vi "TWM Wait for Measure End.vi"(0 "handle":i32, 1 "end of packet key":string="TWM:command:EndOfPacket", 2 "Obtain results? (False)":bool, 3 "timeout [s] (10s)":dbl=30.0, 5 "meas root path (last)":path, 7 "quantity names (all)":string[](array[string]), 9 "stop ref (none)":refnum<vi>, 11 "error in":errorcluster, 12 "qwtb maxdim (scalar)":T3 caption="Max. shown dimension (scalar)", 13 "status ref (none)":refnum<vi>, 14 "phase ref channel tag (none)":string) -> (4 "handle out":i32, 6 "data":T2[][](array[typedef]), 8 "stoped?":bool, 10 "quantities":T1, 15 "error out":errorcluster)   [LabVIEW 2020]
doc: "TWM client top level function: Start measurement, wait for completion, Get result.\n\nSet reasonable timeout for the TWM sampling and processing. Wire in the the 'stop' reference to allow termination of the TWM task."
uses:
  external libraries/TWM client/TWM Client Result Max Dim.ctl
  external libraries/TWM client/TWM Client Quantity Record.ctl
  external libraries/TWM client/TWM Client Result Info.ctl
  <vilib>/Utility/error.llb/Error Cluster From Error Code.vi
  <vilib>/ErrorRing/Error Ring.xnode
  external libraries/TWM client/TWM Client.lvlib
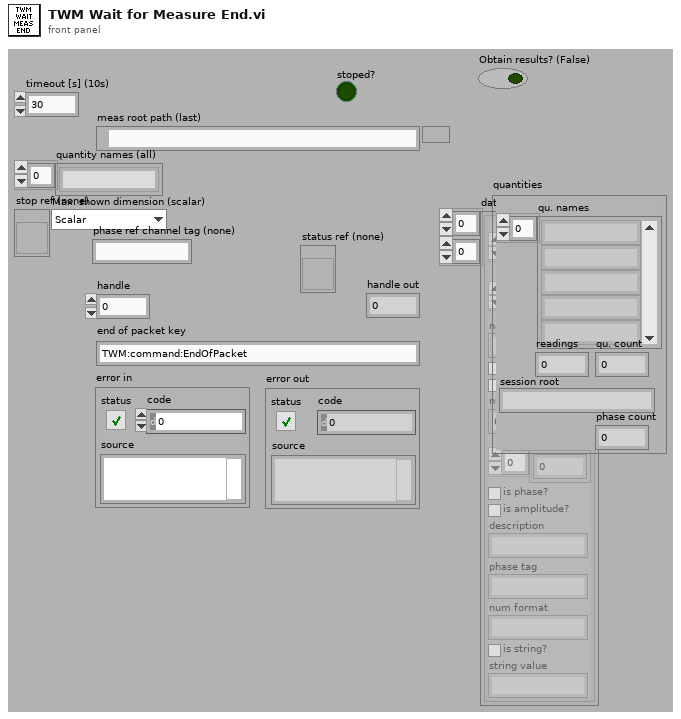
[diagram p1: front panel]
types:
  T1 = typedef "TWM Client.lvlib/TWM Client Result Info.ctl" = cluster{"qu. names":string[], "readings":i32, "qu. count":i32, "session root":string, "phase count":i32}
  T2 = typedef "TWM Client.lvlib/TWM Client Quantity Record.ctl" = cluster{"val":dbl[], "unc":dbl[], "name":string, "is valid?":bool, "has unc?":bool, "numel":i32, "ua":dbl[], "is phase?":bool, "is amplitude?":bool, "description":string, "phase tag":string, "num format":string, "is string?":bool, "string value":string}
  T3 = typedef "TWM Client.lvlib/TWM Client Result Max Dim.ctl" = enum16{"Scalar", "Vector", "Matrix"}
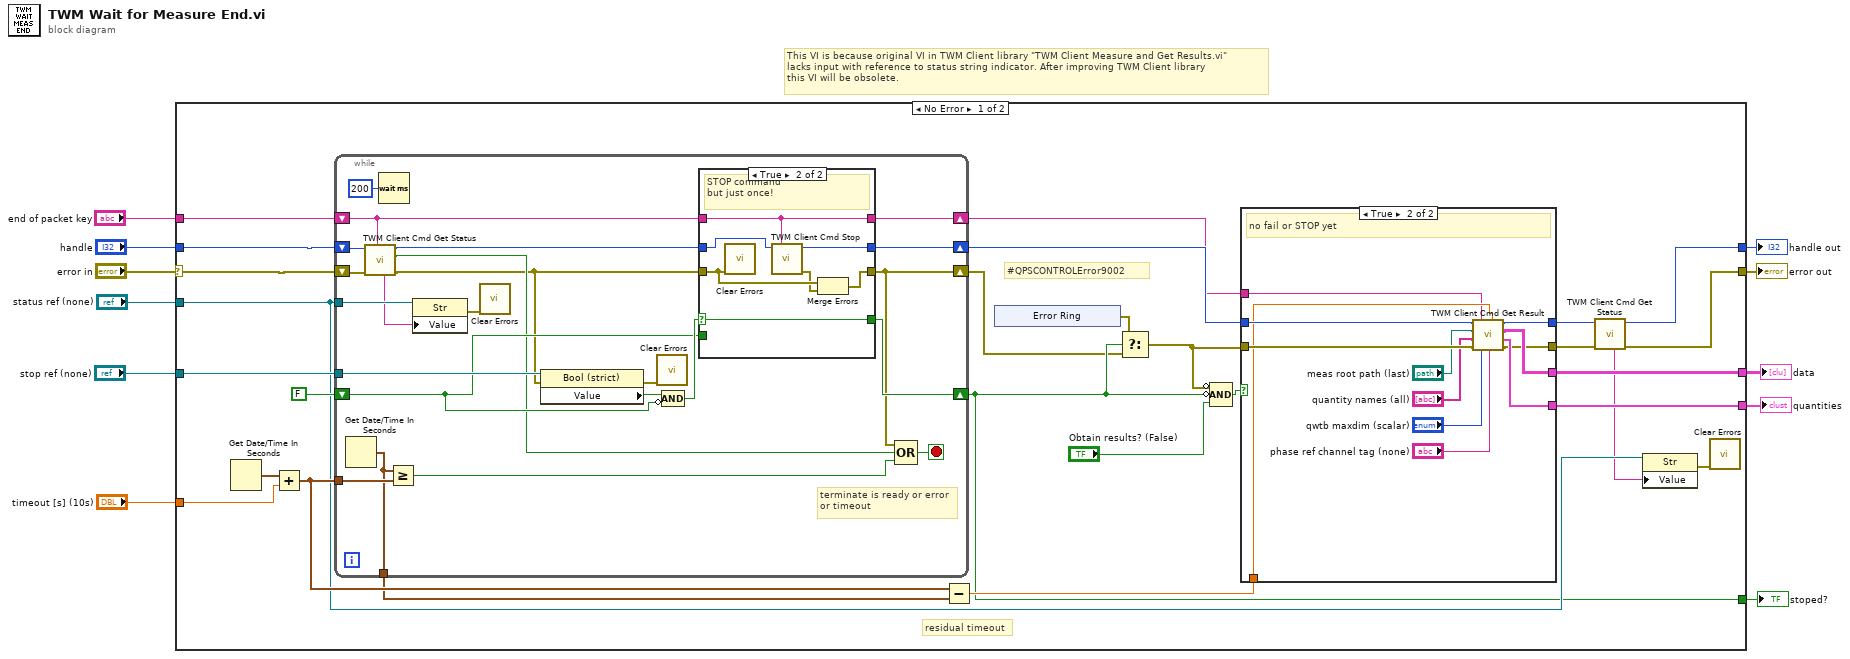
[diagram p0: block diagram]
diagram:
  # "This VI is because original VI in TWM Client library \"TWM Client Measure and Get Results.vi\"\nlacks input with reference to status string indicator. After improving TWM Client library \nthis VI will be obsolete."
  n1 = case shown="No Error" "error in" {
    selector: "error in" -> [w14 w93]
    tunnel: "handle" -> [w13 w92]
    tunnel: "stop ref (none)" -> [w38 _]
    tunnel: "timeout [s] (10s)" -> [w36 _]
    tunnel: "end of packet key" -> [w26 _]
    tunnel: [w24 w92] -> w7
    tunnel: [w22 w93] -> w6
    tunnel: [w28 _] -> w5
    tunnel: [w27 _] -> w4
    tunnel: [w18 _] -> w2
    tunnel: "status ref (none)" -> [w20 _]
    frame No Error {
      # "#QPSCONTROLError9002"
      # "residual timeout"
      n2 = Get Date/Time In Seconds() -> (seconds since 1Jan1904=w35:timestamp)
      n3 = Add(x=w35, y=w36) -> (x+y=w34:timestamp)
      n4 = while {
        shift-right: [w78] -> w31
        shift-left: w13 -> [w62]
        shift-right: [w72] -> w16
        shift-left: w14 -> [w63]
        tunnel: w38 -> [w79]
        shift-right: [w77] -> w18
        shift-left: FALSE -> [w74]
        tunnel: w34 -> [w73]
        tunnel: [w68] -> w33
        shift-right: [w67] -> w29
        shift-left: w26 -> [w61]
        tunnel: w20 -> [w60]
        stop <- w70 stop-if-true
        # "terminate is ready or error\nor timeout"
        n5 = Get Date/Time In Seconds() -> (seconds since 1Jan1904=w68:timestamp)
        n6 = call "TWM Client Cmd Get Status.vi"("end of packet key"=w61, "error in"=w63, "handle"=w62) -> ("error out"=w64:errorcluster, "ready?"=w65:bool, "handle out"=w66:i32, "status string"=w59:string)  [unwired: 4 in, 1 out]
        n7 = Wait (ms)(milliseconds to wait=u32 200) -> ()  [unwired: 1 out]
        n8 = Greater Or Equal?(x=w68, y=w73) -> (x >= y?=w71:bool)
        n9 = property class="Str"(reference=w60, "Value"=w59) -> (error out=w58:errorcluster)  [unwired: 1 in, 1 out]
        n10 = call <vilib>:"Clear Errors.vi"("error in (no error)"=w58) -> ()  [unwired: 5 in, 2 out]
        n11 = property class="Bool (strict)"(reference=w79, error in=w64) -> (error out=w80:errorcluster, "Value"=w76:bool)  [unwired: 1 out]
        n12 = call <vilib>:"Clear Errors.vi"("error in (no error)"=w80) -> ()  [unwired: 5 in, 2 out]
        n13 = Compound Arithmetic op=AND(w76, invert w74) -> (w75:bool)
        n14 = case shown="True" w75 {
          selector: w75 -> [_ w89]
          tunnel: w64 -> [w84 w91]
          tunnel: w66 -> [w83 w86]
          tunnel: [w83 w88] -> w78
          tunnel: [w84 w90] -> w72
          tunnel: [w82 w89] -> w77
          tunnel: w74 -> [w82 _]
          tunnel: w61 -> [w81 w87]
          tunnel: [w81 w87] -> w67
          frame False {
          }
          frame True {
            # "STOP command\nbut just once!"
            n15 = call <vilib>:"Clear Errors.vi"("error in (no error)"=w91) -> ()  [unwired: 5 in, 2 out]
            n16 = call "TWM Client Cmd Stop.vi"("end of packet key"=w87, "handle"=w86) -> ("error out"=w85:errorcluster, "handle out"=w88:i32)  [unwired: 8 in]
            n17 = Merge Errors(w91, w85) -> (w90:errorcluster)
          }
        }
        n18 = Compound Arithmetic op=OR(w72, w65, w71) -> (w70:bool)
      }
      n19 = Subtract(x=w34, y=w33) -> (x-y=w30:dbl)
      n20 = xnode "Error Ring"() -> ("error out"=w15:errorcluster)
      n21 = Select(t=w15, s=w18, f=w16) -> (s? t:f=w17:errorcluster)
      n22 = Compound Arithmetic op=AND(invert w17, invert w18, "Obtain results? (False)") -> (w32:bool)
      n23 = case shown="True" w32 {
        tunnel: w17 -> [w45 w52]
        tunnel: w31 -> [w44 w57]
        tunnel: [w45 w53] -> w23
        tunnel: [w44 w56] -> w25
        tunnel: w30 -> [_ w51]
        tunnel: w29 -> [_ w50]
        tunnel: [_ w55] -> w28
        tunnel: [_ w54] -> w27
        frame False {
          # "STOP or error"
        }
        frame True {
          # "no fail or STOP yet"
          n24 = call "TWM Client Cmd Get Result.vi"("phase ref channel tag (none)"="phase ref channel tag (none)", "timeout [s] (10s)"=w51, "qwtb maxdim (scalar)"="qwtb maxdim (scalar)", "end of packet key"=w50, "error in"=w52, "quantity names (all)"="quantity names (all)", "meas root path (last)"="meas root path (last)", "handle"=w57) -> ("error out"=w53:errorcluster, "result info"=w54:T1, "result data"=w55:T2[][], "handle out"=w56:i32)
        }
      }
      n25 = call "TWM Client Cmd Get Status.vi"("error in"=w23, "handle"=w25) -> ("error out"=w22:errorcluster, "handle out"=w24:i32, "status string"=w19:string)  [unwired: 5 in, 2 out]
      n26 = property class="Str"(reference=w20, "Value"=w19) -> (error out=w21:errorcluster)  [unwired: 1 in, 1 out]
      n27 = call <vilib>:"Clear Errors.vi"("error in (no error)"=w21) -> ()  [unwired: 5 in, 2 out]
    }
    frame Error {
    }
  }
  "error out" <- w6
  "handle out" <- w7
  "data" <- w5
  "quantities" <- w4
  "stoped?" <- w2
